vi "Configure DC Measurement.vi"(7 "Enable DC Measurement (F: Disable)":bool, 8 "error in (no error)":errorcluster, 9 "Measurement Function (0: Vdc Bias)":i32(ring) items=["Vdc Bias", "Idc Bias", "Vdc R", "Vdc T"], 10 "Active Channel (1)":i32=1, 11 "VISA resource name":refnum<visa-resource-name>) -> (0 "error out":errorcluster, 3 "VISA resource name out":refnum<visa-resource-name>)   [LabVIEW 2018, in "Agilent ENA Series.lvlib"]
doc: "Configures the DC output measurement.\n\n<B>Note:</B> This VI is only valid for E5061B."
uses:
  Agilent ENA Series.lvlib
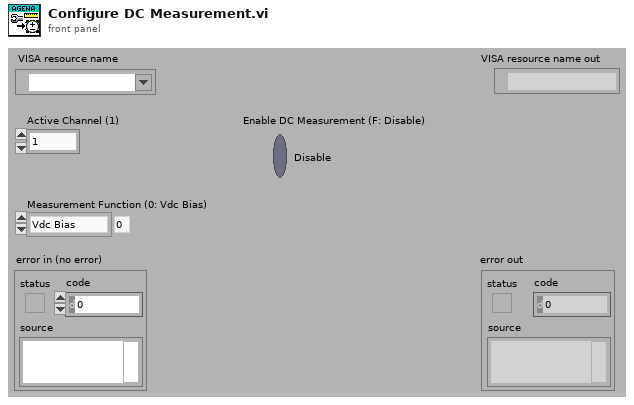
[diagram p1: front panel]
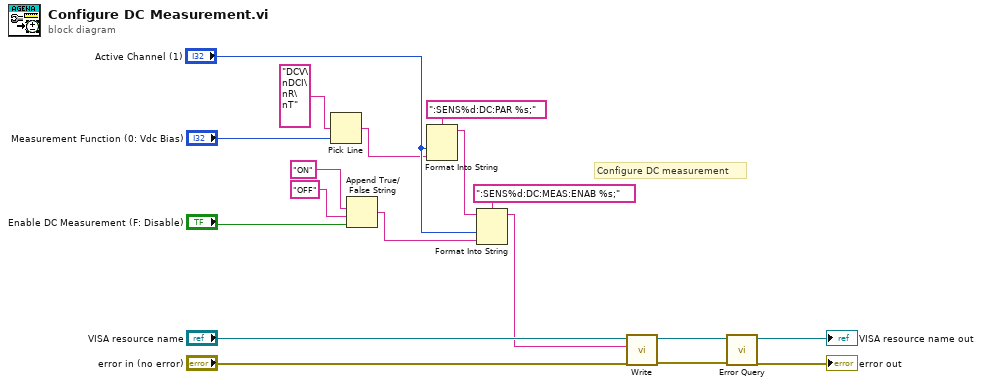
[diagram p0: block diagram]
diagram:
  # "Configure DC measurement"
  n1 = Pick Line(multi-line string="DCV\nDCI\nR\nT", line index="Measurement Function (0: Vdc Bias)") -> (output string=w14:string)  [unwired: 1 out]
  n2 = Append True/False String(1:"Enable DC Measurement (F: Disable)", 2:"OFF", 3:"ON") -> (0:w8:string)  [unwired: 1 out]
  n3 = Format Into String(format string=":SENS%d:DC:PAR %s;", "Active Channel (1)", w14) -> (resulting string=w10:string)  [unwired: 2 in, 1 out]
  n4 = Format Into String(format string=":SENS%d:DC:MEAS:ENAB %s;", initial string=w10, "Active Channel (1)", w8) -> (resulting string=w1:string)  [unwired: 1 in, 1 out]
  n5 = call "Write.vi"("error in (no error)"="error in (no error)", "String ()"=w1, "VISA resource name"="VISA resource name") -> ("error out"=w4:errorcluster, "VISA resource name out"=w5:refnum<visa-resource-name>)  [unwired: 6 in, 1 out]
  n6 = call "Error Query.vi"("error in (no error)"=w4, "VISA resource name"=w5) -> ("error out"=→"error out":errorcluster, "VISA resource name out"=→"VISA resource name out":refnum<visa-resource-name>)  [unwired: 8 out]
